vi "Write Chunk.vi"(8 "error in (no error)":errorcluster, 10 "Content Chunk":string, 11 "Stream in":refnum<k5>) -> (0 "error out":errorcluster, 2 "Done":bool, 3 "Stream out":refnum<k5>)   [LabVIEW 2020, in "HTTP Utils.lvlib" / "Response.lvclass"]
uses:
  Response.lvclass
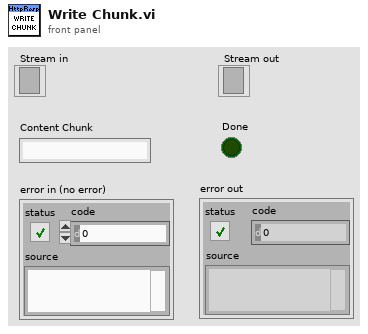
[diagram p1: front panel]
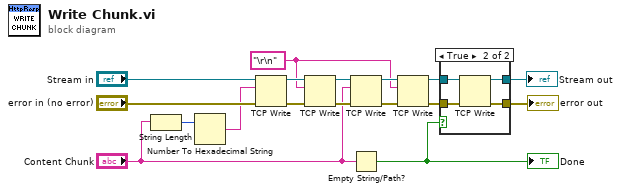
[diagram p0: block diagram]
diagram:
  w1 = "\r\n" ("Data")
  n1 = String Length(string="Content Chunk") -> (length=w17:i32)
  n2 = Number To Hexadecimal String(2:w17) -> (0:w11:string)  [unwired: 1 in]
  n3 = TCP Write(connection ID="Stream in", data in=w11, error in (no error)="error in (no error)") -> (connection ID out=w10:refnum<k5>, error out=w9:errorcluster)  [unwired: 1 in, 1 out]
  n4 = TCP Write(connection ID=w10, data in=w1, error in (no error)=w9) -> (connection ID out=w7:refnum<k5>, error out=w8:errorcluster)  [unwired: 1 in, 1 out]
  n5 = TCP Write(connection ID=w7, data in="Content Chunk", error in (no error)=w8) -> (connection ID out=w3:refnum<k5>, error out=w2:errorcluster)  [unwired: 1 in, 1 out]
  n6 = Empty String/Path?(string/path="Content Chunk") -> (empty?=w14:bool)
  "Done" <- w14
  n7 = TCP Write(connection ID=w3, data in=w1, error in (no error)=w2) -> (connection ID out=w5:refnum<k5>, error out=w4:errorcluster)  [unwired: 1 in, 1 out]
  n8 = case shown="True" w14 {
    tunnel: w4 -> [w19 w22]
    tunnel: w5 -> [w18 w23]
    tunnel: [w18 w21] -> w16
    tunnel: [w19 w20] -> w15
    frame False {
    }
    frame True {
      n9 = TCP Write(connection ID=w23, error in (no error)=w22) -> (connection ID out=w21:refnum<k5>, error out=w20:errorcluster)  [unwired: 2 in, 1 out]
    }
  }
  "Stream out" <- w16
  "error out" <- w15
